vi "_PC_Pub_reg_file_config.vi"(4 "func":enum16{"None", "Write", "Read"}(ring)=enum."Read", 5 "error in (no error)":errorcluster, 6 "FileSN in":dbl, 7 "FileNoise in":dbl, 8 "AutoSave in":bool) -> (0 "error out":errorcluster, 1 "FileSN out":sgl, 2 "FileNoise out":dbl, 3 "AutoSave out":bool)   [LabVIEW 2018]
uses:
  Ctl/RegistyFunc.ctl
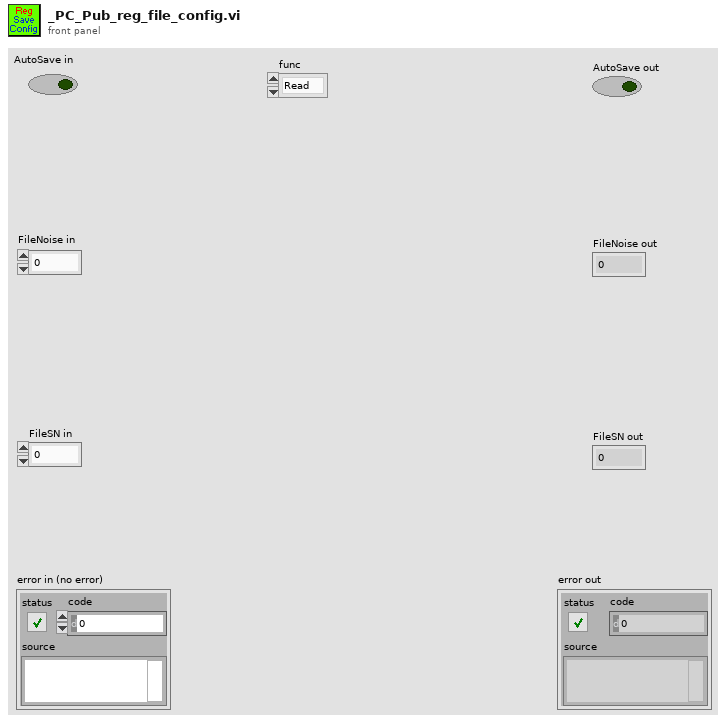
[diagram p1: front panel]
types:
  T1 = typedef "RegistyFunc.ctl" = enum16{"None", "FileAutoSave", "FileNoise", "FileSN", "ExeStatu", "WorkFolderPath", "MethodPath", "AVGItem", "LoopItem", "AutoRun", "BGColor", "LineColor", "LineWidth", "XGrid", "YGrid", "DeviceRefnum"}
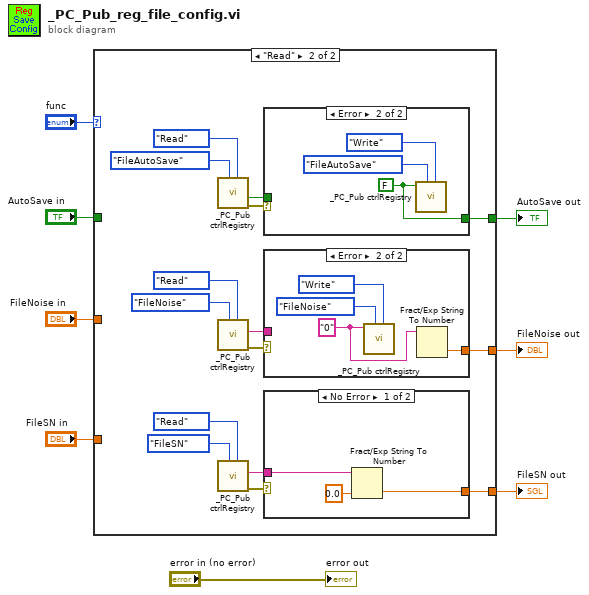
[diagram p0: block diagram]
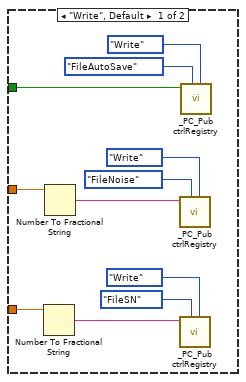
[diagram p2: hidden frame]
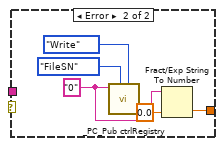
[diagram p3: hidden frame]
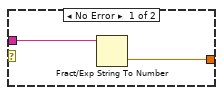
[diagram p4: hidden frame]
diagram:
  n1 = case shown="\"Read\"" "func" {
    tunnel: [_ w30] -> w6
    tunnel: [_ w21] -> w5
    tunnel: "AutoSave in" -> [w13 _]
    tunnel: "FileNoise in" -> [w12 _]
    tunnel: "FileSN in" -> [w11 _]
    tunnel: [_ w20] -> w1
    frame "Write", Default {
      n2 = Number To Fractional String(number=w11) -> (F-format string=w10:string)  [unwired: 3 in]
      n3 = Number To Fractional String(number=w12) -> (F-format string=w9:string)  [unwired: 3 in]
      n4 = call "_PC_Pub ctrlRegistry.vi"("type"=enum16{"None", "Write", "Read"}."Write", "function"=RegistyFunc."FileNoise", "write value"=w9) -> ()  [unwired: 5 in, 4 out]
      n5 = call "_PC_Pub ctrlRegistry.vi"("type"=enum16{"None", "Write", "Read"}."Write", "function"=RegistyFunc."FileSN", "write value"=w10) -> ()  [unwired: 5 in, 4 out]
      n6 = call "_PC_Pub ctrlRegistry.vi"("type"=enum16{"None", "Write", "Read"}."Write", "function"=RegistyFunc."FileAutoSave", "write value"=w13) -> ()  [unwired: 5 in, 4 out]
    }
    frame "Read" {
      n7 = call "_PC_Pub ctrlRegistry.vi"("type"=enum16{"None", "Write", "Read"}."Read", "function"=RegistyFunc."FileAutoSave") -> ("error out"=w32:errorcluster, "Boolean output"=w31:bool)  [unwired: 6 in, 2 out]
      n8 = call "_PC_Pub ctrlRegistry.vi"("type"=enum16{"None", "Write", "Read"}."Read", "function"=RegistyFunc."FileNoise") -> ("error out"=w27:errorcluster, "SZ output"=w24:string)  [unwired: 6 in, 2 out]
      n9 = call "_PC_Pub ctrlRegistry.vi"("type"=enum16{"None", "Write", "Read"}."Read", "function"=RegistyFunc."FileSN") -> ("error out"=w22:errorcluster, "SZ output"=w23:string)  [unwired: 6 in, 2 out]
      n10 = case shown="Error" w32 {
        tunnel: w31 -> [w49 _]
        tunnel: [w49 w50] -> w30
        frame No Error {
        }
        frame Error {
          w50 = FALSE
          n11 = call "_PC_Pub ctrlRegistry.vi"("type"=enum16{"None", "Write", "Read"}."Write", "function"=RegistyFunc."FileAutoSave", "write value"=w50) -> ()  [unwired: 5 in, 4 out]
        }
      }
      n12 = case shown="Error" w27 {
        tunnel: [w43 w45] -> w21
        tunnel: w24 -> [w44 _]
        frame No Error {
          n13 = Fract/Exp String To Number(string=w44) -> (number=w43:dbl)  [unwired: 3 in, 1 out]
        }
        frame Error {
          w46 = "0"
          n14 = call "_PC_Pub ctrlRegistry.vi"("type"=enum16{"None", "Write", "Read"}."Write", "function"=RegistyFunc."FileNoise", "write value"=w46) -> ()  [unwired: 5 in, 4 out]
          n15 = Fract/Exp String To Number(string=w46) -> (number=w45:dbl)  [unwired: 3 in, 1 out]
        }
      }
      n16 = case shown="No Error" w22 {
        tunnel: [w36 w39] -> w20
        tunnel: w23 -> [w37 _]
        frame No Error {
          n17 = Fract/Exp String To Number(string=w37, default (0 dbl)=sgl 0.0 ("default (0 DBL)")) -> (number=w36:sgl)  [unwired: 2 in, 1 out]
        }
        frame Error {
          w40 = "0"
          n18 = call "_PC_Pub ctrlRegistry.vi"("type"=enum16{"None", "Write", "Read"}."Write", "function"=RegistyFunc."FileSN", "write value"=w40) -> ()  [unwired: 5 in, 4 out]
          n19 = Fract/Exp String To Number(string=w40, default (0 dbl)=sgl 0.0 ("default (0 DBL)")) -> (number=w39:sgl)  [unwired: 2 in, 1 out]
        }
      }
    }
  }
  "AutoSave out" <- w6
  "FileNoise out" <- w5
  "FileSN out" <- w1
  "error out" <- "error in (no error)"
